vi "Addressing_sendMultipleCMD.vi"(6 "Address":u16[](array[numeric]), 7 "device_handle":i32, 8 "error in (no error)":errorcluster, 9 "Addressin_Type":T1[](array[typedef]), 10 "Data":u32[](array[numeric]), 11 "Commands":T2[](array[typedef])) -> (0 "error out":errorcluster, 2 "Recieve Answer?":bool)   [LabVIEW 2014, in "Driver_interaction.lvlib" / "Dali_usb_tridonics.lvclass"]
uses:
  Dali_usb_tridonics.lvclass
  Controls/Commands enum.ctl
  Vendor/Controls/Addressing_type.ctl
  Vendor/Dali_usb.lvlib
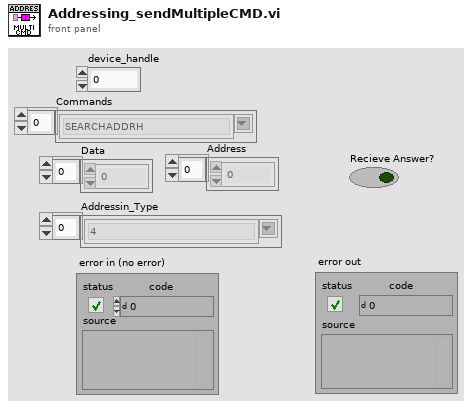
[diagram p1: front panel]
types:
  T1 = typedef "Dali_usb.lvlib/Addressing_type.ctl" = string
  T2 = typedef "Driver_interaction.lvlib/Dali_usb_tridonics.lvclass/Commands enum.ctl" = string
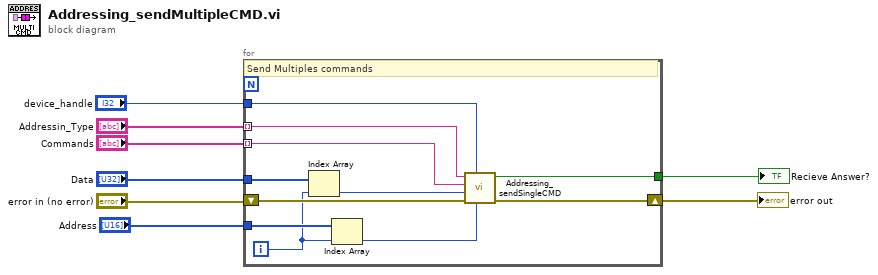
[diagram p0: block diagram]
diagram:
  n1 = for {
    tunnel: "Commands" -> [w19] mode=indexing
    tunnel: "Data" -> [w13]
    tunnel: "Addressin_Type" -> [w18] mode=indexing
    shift-right: [w16] -> w7
    shift-left: "error in (no error)" -> [w17]
    tunnel: [w15] -> w6
    tunnel: "device_handle" -> [w14]
    tunnel: "Address" -> [w11]
    i -> [w10]
    # "Send Multiples commands"
    n2 = Index Array(array=w13, index=w10) -> (element=w12:u32)
    n3 = Index Array(array=w11, index=w10) -> (element=w9:u16)
    n4 = call "Addressing_sendSingleCMD.vi"("address_group"=w9, "device_handle"=w14, "error in (no error)"=w17, "DATA"=w12, "Command"=w19, "addressing_type"=w18) -> ("error out"=w16:errorcluster, "Answer Received?"=w15:bool)  [unwired: 4 in]
  }
  "Recieve Answer?" <- w6
  "error out" <- w7
